vi "Value to Alarm Status.vi"(8 "error in":errorcluster, 11 "value":variant) -> (0 "error out":errorcluster, 1 "Message":string, 2 "Severity":T2(ring), 3 "value out":variant, 5 "Status":T1(ring))   [LabVIEW 2020, in "Value.lvlib"]
uses:
  Value.lvlib
  Alarm Status.ctl
  Alarm Severity.ctl
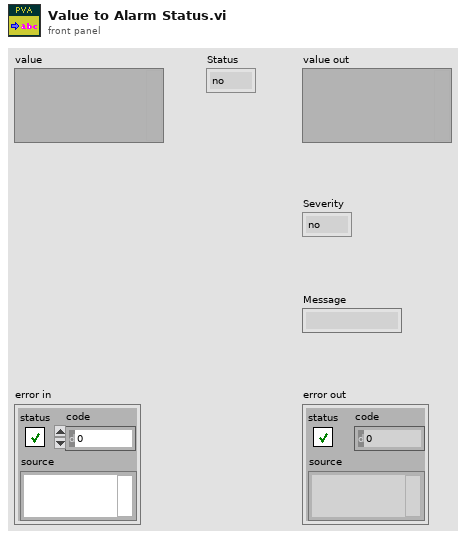
[diagram p1: front panel]
types:
  T1 = enum32{"no", "device", "driver", "record", "db", "conf", "undefined", "client"}
  T2 = enum32{"no", "minor", "major", "record", "invalid", "undefined", ""}
  T3 = typedef "Value.lvlib/Alarm Status.ctl" = cluster{"Severity":T4, "Status":enum32{"no", "device", "driver", "record", "db", "conf", "undefined", "client"}, "Message":string}
  T4 = typedef "Value.lvlib/Alarm Severity.ctl" = enum32{"no", "minor", "major", "record", "invalid", "undefined", ""}
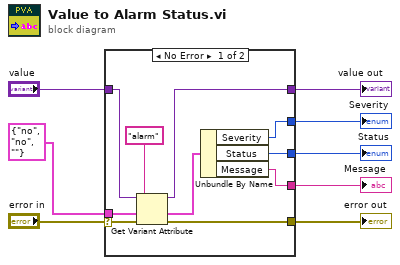
[diagram p0: block diagram]
diagram:
  n1 = case shown="No Error" "error in" {
    selector: "error in" -> [w17 w20]
    tunnel: [w11 w20] -> w8
    tunnel: "value" -> [w18 w19]
    tunnel: [w9 w19] -> w5
    tunnel: T3 {"Severity"=enum."no", "Status"=enum."no", "Message"=""} ("Alarm") -> [w15 _]
    tunnel: [w13 _] -> w3
    tunnel: [w12 _] -> w2
    tunnel: [w10 _] -> w1
    frame No Error {
      n2 = Get Variant Attribute(Variant=w18, name="alarm", default value (empty Variant)=w15, error in=w17) -> (duplicate Variant=w9:variant, value=w14:T3, error out=w11:errorcluster)  [unwired: 1 out]
      n3 = Unbundle By Name(w14) -> ("Severity"=w13:T4, "Status"=w12:T1, "Message"=w10:string)
    }
    frame Error {
    }
  }
  "error out" <- w8
  "value out" <- w5
  "Severity" <- w3
  "Status" <- w2
  "Message" <- w1
